vi "Custom Aggregation.vi"   [LabVIEW 2014, in "NI_EP_Power Quality.lvlib"]
doc: "Calculates the aggregated minimum, maximum, and averaged or RMS value of an input signal for a specified aggregation interval, according to Class S in IEC 61000-4-30:2008. There is no overlap between aggregation intervals. This VI automatically restarts accumulation at the beginning of the next time interval after the previous interval expires. You must manually select the polymorphic instance you want to use.\n\nThis VI supports measuring single-line and multiple-line systems except the DBL instance. Use the DBL instance to measure one channel on one line at one time."
uses:
  <vilib>/addons/Electrical Power/PQ/NI_EP_Power Quality.lvlib
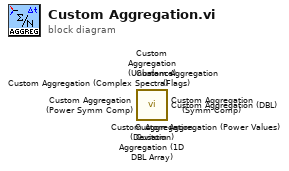
[diagram p0: block diagram]
diagram:
  n1 = call <vilib>:"Custom Aggregation (Deviation).vi"() -> ()  [unwired: 10 in, 6 out]
  n2 = call <vilib>:"Custom Aggregation (Flags).vi"() -> ()  [unwired: 11 in, 5 out]
  n3 = call <vilib>:"Custom Aggregation (Power Symm Comp).vi"() -> ()  [unwired: 9 in, 7 out]
  n4 = call <vilib>:"Custom Aggregation (Symm Comp).vi"() -> ()  [unwired: 9 in, 7 out]
  n5 = call <vilib>:"Custom Aggregation (Complex Spectra).vi"() -> ()  [unwired: 9 in, 7 out]
  n6 = call <vilib>:"Custom Aggregation (Unbalance).vi"() -> ()  [unwired: 9 in, 7 out]
  n7 = call <vilib>:"Custom Aggregation (Power Values).vi"() -> ()  [unwired: 9 in, 7 out]
  n8 = call <vilib>:"Custom Aggregation (1D DBL Array).vi"() -> ()  [unwired: 9 in, 7 out]
  n9 = call <vilib>:"Custom Aggregation (DBL).vi"() -> ()  [unwired: 9 in, 7 out]
